vi "boolean.vi"() -> ()   [LabVIEW 2024]
panel:
  out "NOT 6":bool
  out "NAND":bool
  out "X-OR":bool
  out "OR":bool
  out "AND":bool
  in  "Boolean 2":bool
  in  "Boolean":bool
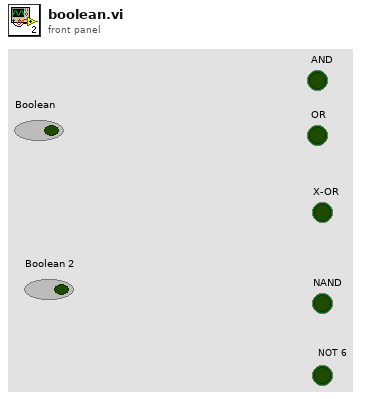
[diagram p1: front panel]
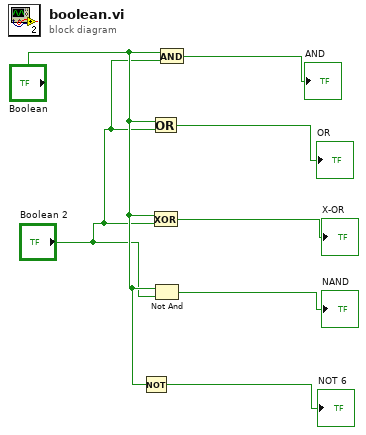
[diagram p0: block diagram]
diagram:
  n1 = Not(x="Boolean") -> (.not. x?=→"NOT 6":bool)
  n2 = Or(x="Boolean", y="Boolean 2") -> (x .or. y?=→"OR":bool)
  n3 = Exclusive Or(1:"Boolean 2", 2:"Boolean") -> (0:→"X-OR":bool)
  n4 = Not And(1:"Boolean 2", 2:"Boolean") -> (0:→"NAND":bool)
  n5 = And(x="Boolean", y="Boolean 2") -> (x .and. y?=→"AND":bool)
